vi "Slide-Control_Api.vi"(8 "Error In":errorcluster, 11 "狀態選擇":enum16{"重置", "下降"}(ring)) -> (0 "Error Out":errorcluster)   [LabVIEW 2019]
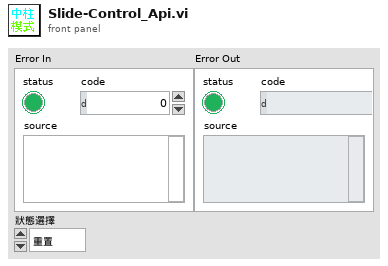
[diagram p1: front panel]
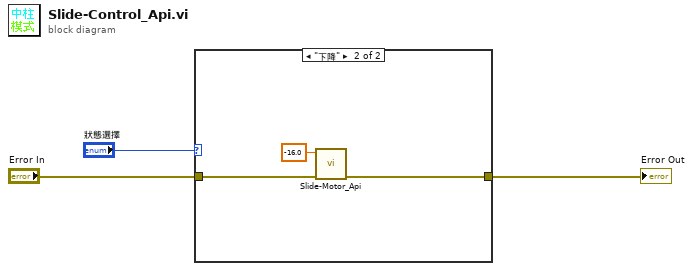
[diagram p0: block diagram]
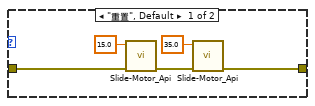
[diagram p2: hidden frame]
diagram:
  n1 = case shown="\"下降\"" "狀態選擇" {
    tunnel: "Error In" -> [w8 w11]
    tunnel: [w4 w10] -> w2
    frame "重置", Default {
      n2 = call "Slide-Motor_Api.vi"("Error In"=w8, "移動距離"=15.0) -> ("Error Out"=w7:errorcluster)  [unwired: 9 in]
      n3 = call "Slide-Motor_Api.vi"("Error In"=w7, "移動距離"=35.0) -> ("Error Out"=w4:errorcluster)  [unwired: 9 in]
    }
    frame "下降" {
      n4 = call "Slide-Motor_Api.vi"("Error In"=w11, "移動距離"=-16.0) -> ("Error Out"=w10:errorcluster)  [unwired: 9 in]
    }
  }
  "Error Out" <- w2
